vi "Apply Pressure Offset.vi"(9 "Pressure Offset":dbl format="%#_13g", 10 "Untorn Pressure":dbl format="%#_13g") -> (2 "Torn Pressure":dbl)   [LabVIEW 2019]
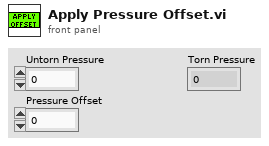
[diagram p1: front panel]
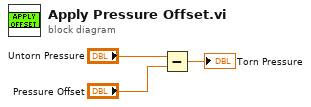
[diagram p0: block diagram]
diagram:
  n1 = Subtract(x="Untorn Pressure", y="Pressure Offset") -> (x-y=→"Torn Pressure":dbl)
